vi "ep_Check Samples Per Cycle.vi"(8 "error in (no error)":errorcluster, 11 "samples per cycle":u16) -> (0 "error out":errorcluster, 3 "dup samples per cycle":u16)   [LabVIEW 2013, in "NI_EP_Power Measurement.lvlib"]
uses:
  <vilib>/addons/Electrical Power/Power Measurement/NI_EP_Power Measurement.lvlib
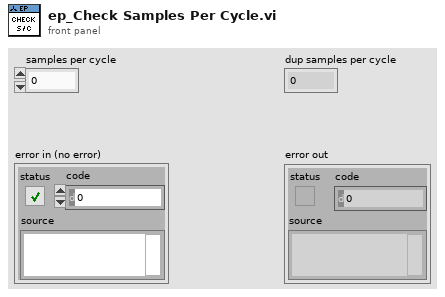
[diagram p1: front panel]
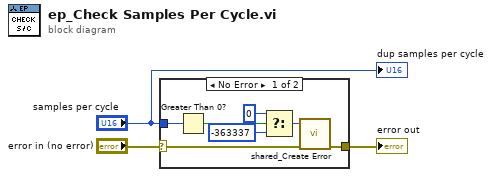
[diagram p0: block diagram]
diagram:
  n1 = case shown="No Error" "error in (no error)" {
    selector: "error in (no error)" -> [w6 w11]
    tunnel: "samples per cycle" -> [w7 _]
    tunnel: [w4 w11] -> w2
    frame No Error {
      n2 = Greater Than 0?(x=w7) -> (x > 0?=w9:bool)
      n3 = Select(t=0 ("error code (0)"), s=w9, f=-363337 ("error code (0)")) -> (s? t:f=w8:i32)
      n4 = call <vilib>:"shared_Create Error.vi"("error in (no error)"=w6, "error code (0)"=w8) -> ("error out"=w4:errorcluster)  [unwired: 9 in]
    }
    frame Error {
    }
  }
  "error out" <- w2
  "dup samples per cycle" <- "samples per cycle"
